vi "Get sequence list.vi"(1 "all rows":string[][](array[string])) -> (0 "Output sequence":T1[](array[typedef]))   [LabVIEW 2020]
uses:
  Control/Setup - Sequence Data.ctl
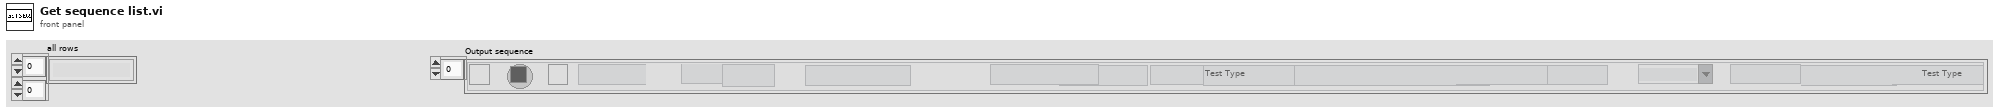
[diagram p1: front panel]
types:
  T1 = typedef "Setup - Sequence Data.ctl" = cluster{"Seq.Select":bool, "Seq.Status":u32, "Seq.Run":bool, "Seq.TestSequence":string, "Seq.No":string, "Seq.ReqID":string, "Seq.TestReq":string, "Seq.Variance":string, "Seq.TestProcedure":string, "Seq.Section":string, "Seq.TestBunker":string, "Seq.TestMedia":string, "Seq.TestPressure":string, "Seq.Cycle":string, "Seq.HoldingTime":string, "Seq.ChartScale":string, "Seq.BDIndicator":string, "Seq.ActuatorPressure":string, "Seq.MaxBDPressure":string}
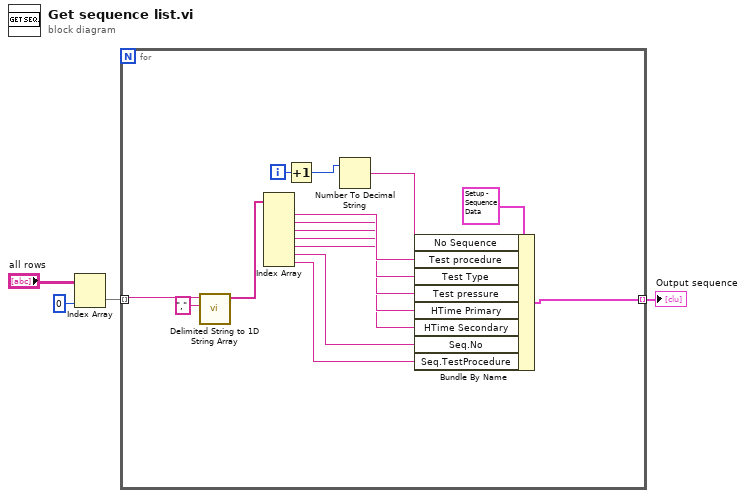
[diagram p0: block diagram]
diagram:
  n1 = Index Array(array="all rows", index (col)=0 ("disabled index (col)")) -> (element=w2:string[])  [unwired: 1 in]
  n2 = for {
    tunnel: w2 -> [w19] mode=indexing
    tunnel: [w5] -> w1 mode=indexing
    i -> [w15]
    n3 = call <vilib>:"Delimited String to 1D String Array.vi"("delimiter"=",", "delimited string"=w19) -> ("string array"=w17:string[])  [unwired: 9 in]
    n4 = Index Array(array=w17) -> (element #1=w12:string, element #2=w11:string, element #3=w10:string, element #4=w9:string, element #5=w8:string, element #6=w7:string, element #7=w6:string)  [unwired: 7 in]
    n5 = Increment(x=w15) -> (x+1=w14:i32)
    n6 = Number To Decimal String(number=w14) -> (decimal integer string=w13:string)  [unwired: 1 in]
    n7 = Bundle By Name(cluster=T1 {"Seq.Select"=FALSE, "Seq.Status"=0, "Seq.Run"=FALSE, "Seq.TestSequence"="", "Seq.No"="", "Seq.ReqID"="", "Seq.TestReq"="", "Seq.Variance"="", "Seq.TestProcedure"="", "Seq.Section"="", "Seq.TestBunker"="Test Type", "Seq.TestMedia"="", "Seq.TestPressure"="", "Seq.Cycle"="", "Seq.HoldingTime"="", "Seq.ChartScale"="", "Seq.BDIndicator"="", "Seq.ActuatorPressure"="", "Seq.MaxBDPressure"="Test Type"} ("Setup - Sequence Data"), "No Sequence"=w13, "Test procedure"=w12, "Test Type"=w11, "Test pressure"=w10, "HTime Primary"=w9, "HTime Secondary"=w8, "Seq.No"=w7, "Seq.TestProcedure"=w6) -> (w5:T1)
  }
  "Output sequence" <- w1
